vi "Auto Pike.vi"(9 "Pike Command":dbl) -> ()   [LabVIEW 2014]
uses:
  Pike/Pike Command.ctl
  Pike/Pike Mode.ctl
  Robot Global Data.vi
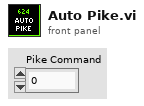
[diagram p1: front panel]
types:
  T1 = typedef "Pike Command.ctl" = cluster{"Command":T2}
  T2 = typedef "Pike Mode.ctl" = enum16{"Idle", "Auto Down", "Auto Up", "Manual Down", "Manual Up"}
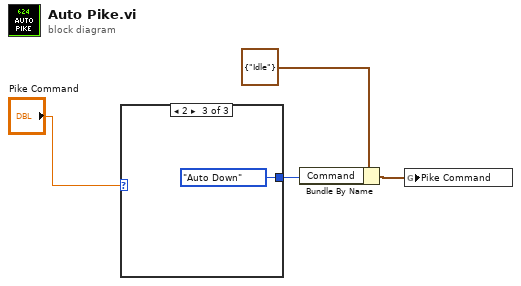
[diagram p0: block diagram]
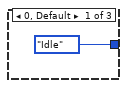
[diagram p2: hidden frame]
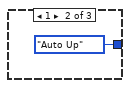
[diagram p3: hidden frame]
diagram:
  n1 = case shown="2" "Pike Command" {
    tunnel: [Pike_Mode."Idle" ("Command") Pike_Mode."Auto Up" ("Command") Pike_Mode."Auto Down" ("Command")] -> w1
    frame 0, Default {
    }
    frame 1 {
    }
    frame 2 {
    }
  }
  n2 = Bundle By Name(cluster=T1 {"Command"=enum."Idle"} ("Pike Command"), "Command"=w1) -> (w2:T1)
  n3 = global write "Robot Global Data.vi" "Pike Command"(w2) -> ()
